vi "DAOUT.vi"(7 "maxInitial数组":i32[](array[numeric]), 8 "maxInitialVoltage":dbl, 9 "changeSymbol":dbl, 10 "running recycle counter":i32, 11 "compensate":dbl) -> (0 "jump symbol":bool, 2 "real running DA output":dbl)   [LabVIEW 2018]
panel:
  out "max Jumped stable boolean":bool
  out "should DA output":dbl
  out "min Jumping booeanl":bool
  out "max Jumping boolean":bool
  out "min output Jump":dbl
  out "max output Jump":dbl
  out "max完全补偿average":dbl
  out "min完全补偿average":dbl
  out "含补偿max理应在偏差范围内":bool
  out "含补偿min理应在偏差范围内":bool
  out "max jump status array output":dbl[](array[numeric])
  out "min jump status array output":dbl[](array[numeric])
  out "min total jump value":dbl
  out "max total jump value":dbl
  out "min Jumped stable boolean":bool
  out "min jumping status output":dbl[](array[numeric])
  out "max jumping status output":dbl[](array[numeric])
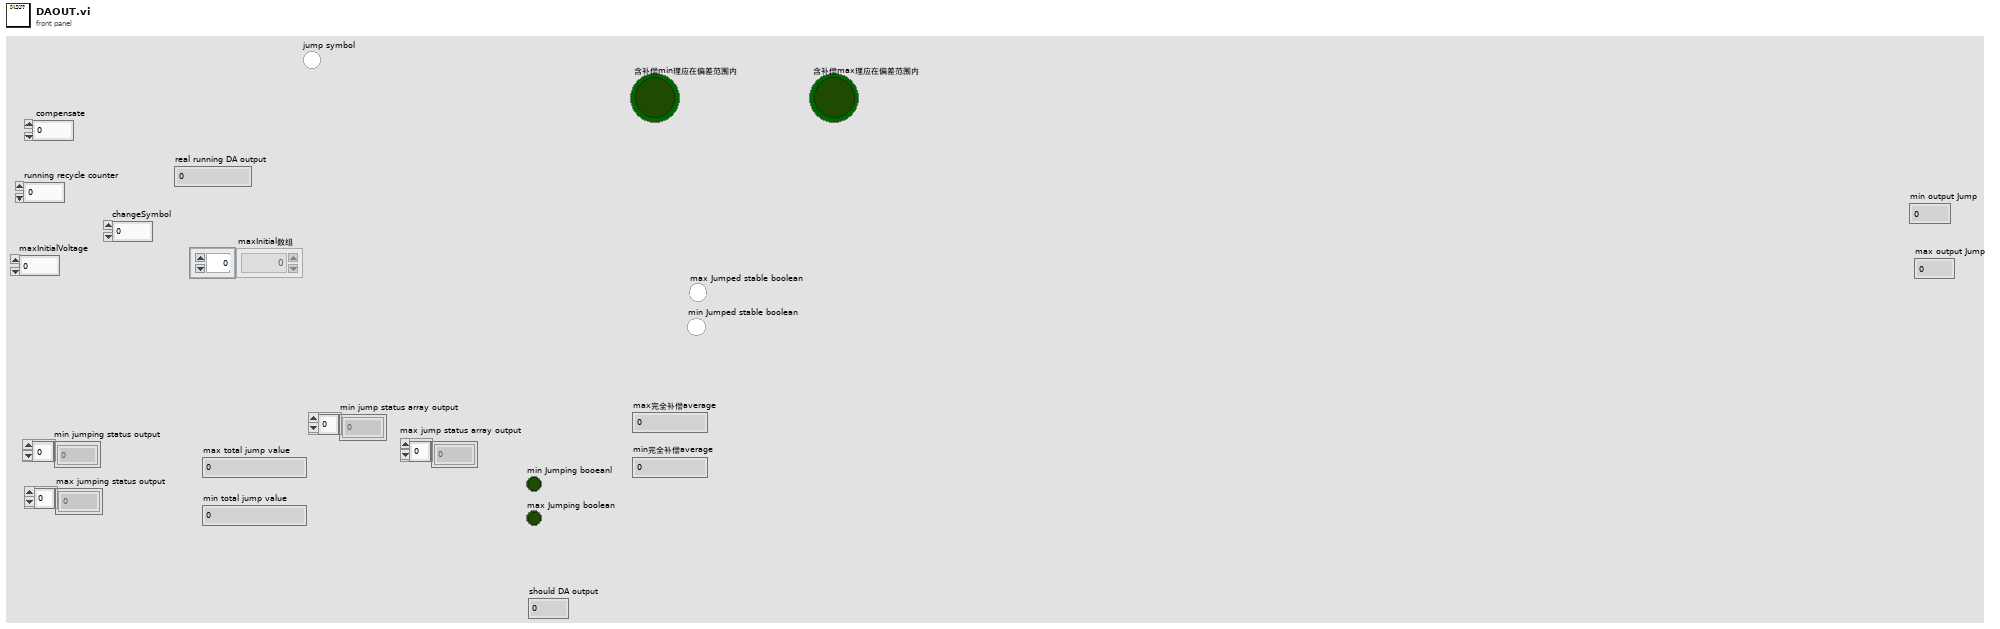
[diagram p1: front panel]
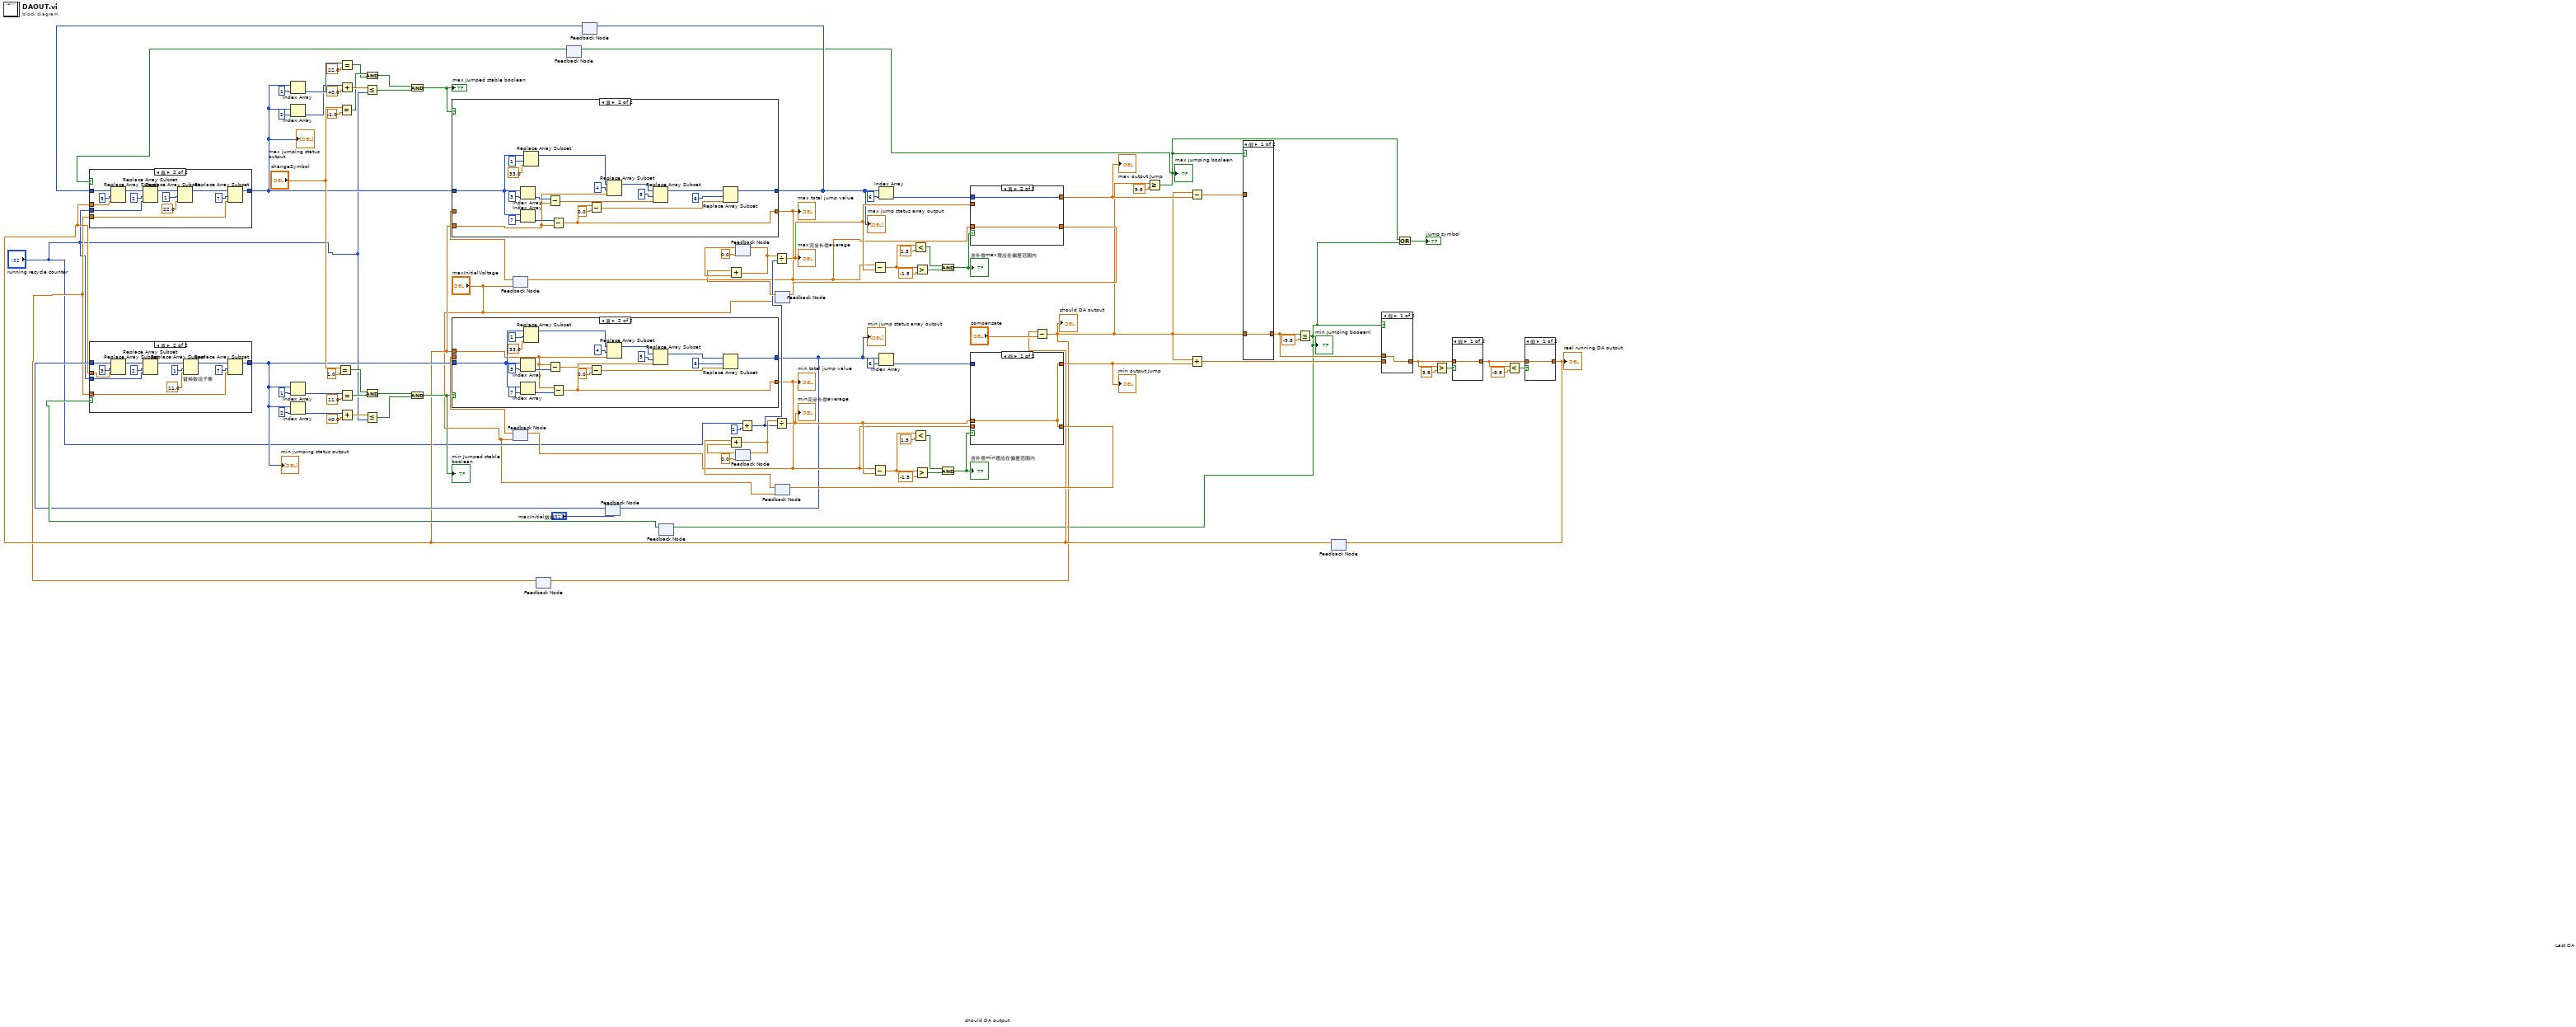
[diagram p0: block diagram]
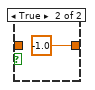
[diagram p2: hidden frame]
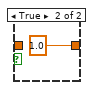
[diagram p3: hidden frame]
diagram:
  n1 = Equal?(x="changeSymbol", y=1.0) -> (x = y?=w84:bool)
  n2 = Equal?(x="changeSymbol", y=-1.0) -> (x = y?=w72:bool)
  n3 = feedback #1("maxInitialVoltage") -> (w68:dbl)
  n4 = feedback #2("maxInitialVoltage") -> (w67:dbl)
  n5 = feedback #3 "should DA output"() -> (w7:dbl)  [unwired: 1 in]
  n6 = feedback #4() -> (w15:bool)  [unwired: 1 in]
  n7 = feedback #5() -> (w11:i32[])  [unwired: 1 in]
  n8 = feedback #6("maxInitial数组") -> (w13:i32[])
  n9 = feedback #7() -> (w16:bool)  [unwired: 1 in]
  n10 = feedback #8(0.0) -> (w56:dbl)
  n11 = feedback #9(0.0) -> (w53:dbl)
  n12 = Add(x="running recycle counter", y=1) -> (x+y=w42:i32)
  n13 = feedback #10("maxInitialVoltage") -> (w49:dbl)
  n14 = Add(x=w49, y=w56) -> (x+y=w57:dbl)
  n15 = feedback-in #8(w57) -> ()
  n16 = Divide(x=w57, y=w42) -> (x/y=w41:dbl)
  "max完全补偿average" <- w41
  n17 = feedback #11("maxInitialVoltage") -> (w47:dbl)
  n18 = Add(x=w47, y=w53) -> (x+y=w54:dbl)
  n19 = feedback-in #9(w54) -> ()
  n20 = Divide(x=w54, y=w42) -> (x/y=w44:dbl)
  "min完全补偿average" <- w44
  n21 = feedback #12 "Last DA"() -> (w9:dbl)  [unwired: 1 in]
  n22 = case shown="真" w15 {
    tunnel: w11 -> [w94 w101]
    tunnel: w9 -> [_ w100]
    tunnel: "running recycle counter" -> [_ w99]
    tunnel: [w94 w97] -> w26
    tunnel: w7 -> [_ w95]
    frame False {
    }
    frame True {
      n23 = Replace Array Subset(array=w101, new element=w100, index=3 ("索引")) -> (w105:i32[])
      n24 = Replace Array Subset(array=w105, new element=w99, index=2 ("索引")) -> (w104:i32[])
      n25 = Replace Array Subset(array=w104, new element=22.0 ("新元素/子数组"), index=1 ("索引")) -> (w96:i32[])
      n26 = Replace Array Subset(array=w96, new element=w95, index=7 ("索引")) -> (w97:i32[])
    }
  }
  "max jumping status output" <- w26
  n27 = case shown="真" w16 {
    tunnel: w13 -> [w108 w115]
    tunnel: w9 -> [_ w114]
    tunnel: "running recycle counter" -> [_ w113]
    tunnel: [w108 w109] -> w25
    tunnel: w7 -> [_ w111]
    frame False {
    }
    frame True {
      n28 = Replace Array Subset(array=w115, new element=w114, index=3 ("索引")) -> (w119:i32[])
      n29 = Replace Array Subset(array=w119, new element=w113, index=2 ("索引")) -> (w118:i32[])
      n30 = Replace Array Subset "替换数组子集"(array=w118, new element=11.0 ("新元素/子数组"), index=1 ("索引")) -> (w110:i32[])
      n31 = Replace Array Subset(array=w110, new element=w111, index=7 ("索引")) -> (w109:i32[])
    }
  }
  "min jumping status output" <- w25
  n32 = Index Array(array=w26, index=1 ("索引")) -> (element=w80:i32)
  n33 = Index Array(array=w26, index=2 ("索引")) -> (element=w77:i32)
  n34 = Index Array(array=w25, index=1 ("索引")) -> (element=w92:i32)
  n35 = Index Array(array=w25, index=2 ("索引")) -> (element=w89:i32)
  n36 = Equal?(x=w80, y=22.0) -> (x = y?=w71:bool)
  n37 = Add(x=w77, y=40.0) -> (x+y=w75:dbl)
  n38 = Equal?(x=w92, y=11.0) -> (x = y?=w83:bool)
  n39 = Add(x=w89, y=40.0) -> (x+y=w87:dbl)
  n40 = Less Or Equal?(x=w75, y="running recycle counter") -> (x <= y?=w74:bool)
  n41 = Less Or Equal?(x=w87, y="running recycle counter") -> (x <= y?=w86:bool)
  n42 = And(x=w72, y=w71) -> (x .and. y?=w70:bool)
  n43 = And(x=w84, y=w83) -> (x .and. y?=w82:bool)
  n44 = And(x=w70, y=w74) -> (x .and. y?=w28:bool)
  "max Jumped stable boolean" <- w28
  n45 = And(x=w82, y=w86) -> (x .and. y?=w27:bool)
  "min Jumped stable boolean" <- w27
  n46 = case shown="真" w28 {
    tunnel: w26 -> [w123 w129]
    tunnel: w9 -> [_ w127]
    tunnel: [w123 w124] -> w12
    tunnel: [w122 w126] -> w24
    tunnel: w68 -> [w122 _]
    frame False {
    }
    frame True {
      n47 = Index Array(array=w129, index=3 ("索引")) -> (element=w133:i32)
      n48 = Index Array(array=w129, index=7 ("索引")) -> (element=w128:i32)
      n49 = Replace Array Subset(array=w129, new element=33.0 ("新元素/子数组"), index=1 ("索引")) -> (w139:i32[])
      n50 = Subtract(x=w133, y=w127) -> (x-y=w132:dbl)
      n51 = Subtract(x=w128, y=w127) -> (x-y=w126:dbl)
      n52 = Subtract(x=w126, y=0.0) -> (x-y=w125:dbl)
      n53 = Replace Array Subset(array=w139, new element=w127, index=4 ("索引")) -> (w136:i32[])
      n54 = Replace Array Subset(array=w136, new element=w132, index=5 ("索引")) -> (w135:i32[])
      n55 = Replace Array Subset(array=w135, new element=w125, index=6 ("索引")) -> (w124:i32[])
    }
  }
  "max total jump value" <- w24
  "max jump status array output" <- w12
  n56 = case shown="真" w27 {
    tunnel: w25 -> [w144 w148]
    tunnel: w9 -> [_ w146]
    tunnel: [w144 w155] -> w14
    tunnel: [w143 w145] -> w23
    tunnel: w67 -> [w143 _]
    frame False {
    }
    frame True {
      n57 = Index Array(array=w148, index=3 ("索引")) -> (element=w162:i32)
      n58 = Index Array(array=w148, index=7 ("索引")) -> (element=w147:i32)
      n59 = Replace Array Subset(array=w148, new element=33.0 ("新元素/子数组"), index=1 ("索引")) -> (w159:i32[])
      n60 = Subtract(x=w146, y=w162) -> (x-y=w152:dbl)
      n61 = Subtract(x=w146, y=w147) -> (x-y=w145:dbl)
      n62 = Subtract(x=w145, y=0.0) -> (x-y=w150:dbl)
      n63 = Replace Array Subset(array=w159, new element=w146, index=4 ("索引")) -> (w156:i32[])
      n64 = Replace Array Subset(array=w156, new element=w152, index=5 ("索引")) -> (w154:i32[])
      n65 = Replace Array Subset(array=w154, new element=w150, index=6 ("索引")) -> (w155:i32[])
    }
  }
  "min total jump value" <- w23
  "min jump status array output" <- w14
  n66 = feedback-in #1(w24) -> ()
  n67 = feedback-in #2(w23) -> ()
  n68 = feedback-in #5(w12) -> ()
  n69 = feedback-in #6(w14) -> ()
  n70 = Subtract(x=w24, y=w41) -> (x-y=w55:dbl)
  n71 = Subtract(x=w23, y=w44) -> (x-y=w48:dbl)
  n72 = Index Array(array=w12, index=6 ("索引")) -> (element=w19:i32)
  n73 = Index Array(array=w14, index=6 ("索引")) -> (element=w20:i32)
  n74 = Less?(x=w55, y=1.5) -> (x < y?=w64:bool)
  n75 = Less?(x=w48, y=1.5) -> (x < y?=w66:bool)
  n76 = Greater?(x=w55, y=-1.5) -> (0:w63:bool)
  n77 = Greater?(x=w48, y=-1.5) -> (0:w65:bool)
  n78 = And(x=w64, y=w63) -> (x .and. y?=w50:bool)
  "含补偿max理应在偏差范围内" <- w50
  n79 = And(x=w66, y=w65) -> (x .and. y?=w58:bool)
  "含补偿min理应在偏差范围内" <- w58
  n80 = case shown="真" w50 {
    tunnel: [w164 w165] -> w17
    tunnel: [w164 w166] -> w45
    tunnel: w24 -> [_ w166]
    tunnel: w41 -> [w164 _]
    tunnel: w19 -> [_ w165]
    frame False {
    }
    frame True {
    }
  }
  "max output Jump" <- w17
  n81 = feedback-in #10(w45) -> ()
  n82 = case shown="假" w58 {
    tunnel: w20 -> [_ w169]
    tunnel: [w167 w169] -> w18
    tunnel: w44 -> [w167 _]
    tunnel: w23 -> [_ w168]
    tunnel: [w167 w168] -> w46
    frame False {
    }
    frame True {
    }
  }
  "min output Jump" <- w18
  n83 = feedback-in #11(w46) -> ()
  n84 = Subtract(x=w9, y="compensate") -> (x-y=w8:dbl)
  "should DA output" <- w8
  n85 = feedback-in #3(w8) -> ()
  n86 = Greater Or Equal?(x=w8, y=9.8) -> (x >= y?=w3:bool)
  "max Jumping boolean" <- w3
  n87 = feedback-in #4(w3) -> ()
  n88 = Subtract(x=w8, y=w17) -> (x-y=w40:dbl)
  n89 = Add(x=w8, y=w18) -> (x+y=w39:dbl)
  n90 = case shown="假" w3 {
    tunnel: w8 -> [w170 _]
    tunnel: [w170 w171] -> w38
    tunnel: w40 -> [_ w171]
    frame False {
    }
    frame True {
    }
  }
  n91 = Less Or Equal?(x=w38, y=-9.8) -> (x <= y?=w2:bool)
  "min Jumping booeanl" <- w2
  n92 = feedback-in #7(w2) -> ()
  n93 = case shown="假" w2 {
    tunnel: [w172 w173] -> w29
    tunnel: w38 -> [w172 _]
    tunnel: w39 -> [_ w173]
    frame False {
    }
    frame True {
    }
  }
  n94 = Or(x=w3, y=w2) -> (x .or. y?=→"jump symbol":bool)
  n95 = Greater?(x=w29, y=9.8) -> (0:w33:bool)
  n96 = case shown="假" w33 {
    tunnel: w29 -> [w174 _]
    tunnel: [w174 1.0] -> w30
    frame False {
    }
    frame True {
    }
  }
  n97 = Less?(x=w30, y=-9.8) -> (x < y?=w31:bool)
  n98 = case shown="假" w31 {
    tunnel: [w176 -1.0] -> w10
    tunnel: w30 -> [w176 _]
    frame False {
    }
    frame True {
    }
  }
  "real running DA output" <- w10
  n99 = feedback-in #12(w10) -> ()
